vi "Cancel State Machine.vi"   [LabVIEW 2013]
uses:
  typedefs/fg_typedef.ctl
  typedefs/subStates.ctl
  typedefs/singleUseSubstate.ctl
types:
  T1 = typedef "subStates.ctl" = enum16{"null", "wait", "driver control", "auto", "manual override", "hold position", "rotate", "pickup", "pass", "load-shoot", "load-pass", "goto shoot", "shoot", "cancel", "end"}
  T2 = typedef "fg_typedef.ctl" = enum16{"Get", "Set"}
  T3 = typedef "singleUseSubstate.ctl" = enum16{"null", "wait", "shift high", "shift low", "extend shooter", "retract shooter", "close latch", "open latch"}
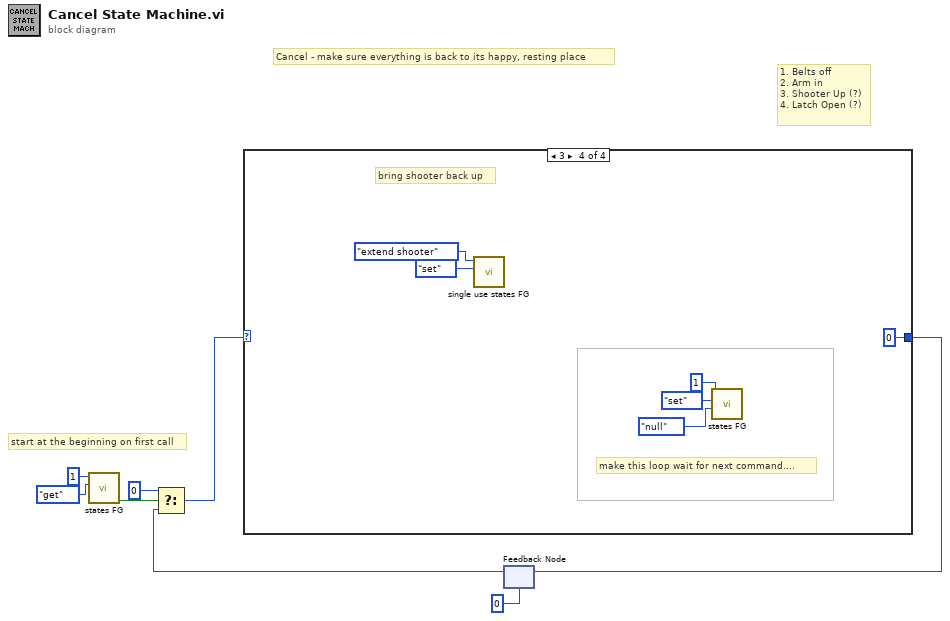
[diagram p0: block diagram]
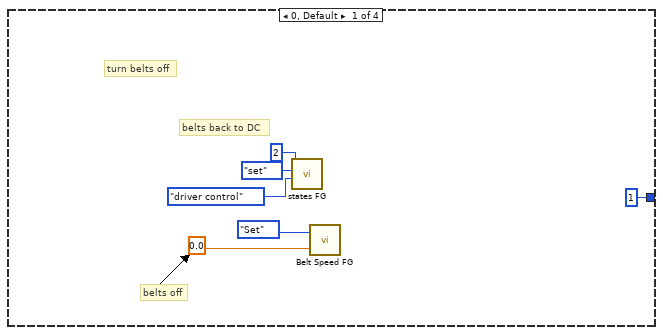
[diagram p2: hidden frame]
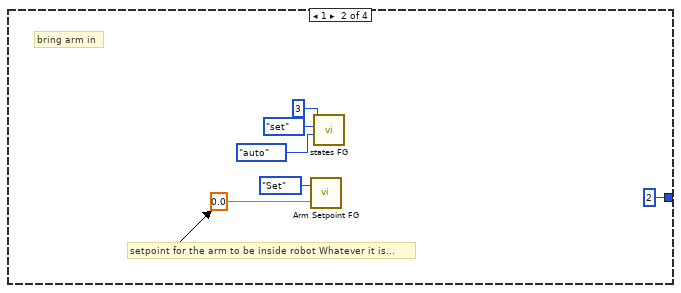
[diagram p3: hidden frame]
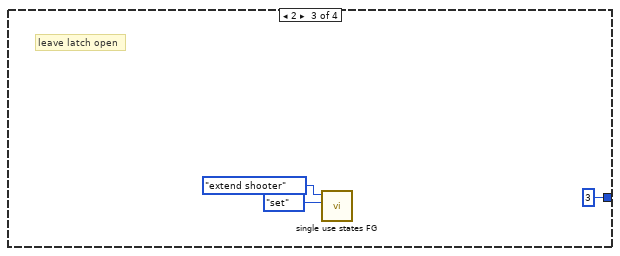
[diagram p4: hidden frame]
diagram:
  # "start at the beginning on first call"
  # "1. Belts off\n2. Arm in\n3. Shooter Up (?)\n4. Latch Open (?)"
  # "Cancel - make sure everything is back to its happy, resting place"
  n1 = call "states FG.vi"("menu (get)"=enum16{"set", "get"}."get", "Loop ID"=1) -> ("first call?"=w1:bool)  [unwired: 6 in, 3 out]
  n2 = feedback #1(0) -> (w4:i32)
  n3 = Select(t=0, s=w1, f=w4) -> (s? t:f=w3:i32)
  n4 = case shown="3" w3 {
    tunnel: [1 2 3 0] -> w7
    frame 0, Default {
      # "belts back to DC"
      # "belts off"
      # "turn belts off"
      n5 = call "states FG.vi"("subState in"=subStates."driver control", "menu (get)"=enum16{"set", "get"}."set", "Loop ID"=2) -> ()  [unwired: 5 in, 4 out]
      n6 = call "Belt Speed FG.vi"("Speed In"=0.0 ("Setpoint In"), "Menu"=fg_typedef."Set") -> ()  [unwired: 1 out]
    }
    frame 1 {
      # "setpoint for the arm to be inside robot Whatever it is..."
      # "bring arm in"
      n7 = call "Arm Setpoint FG.vi"("Setpoint In"=0.0, "Menu"=fg_typedef."Set") -> ()  [unwired: 1 out]
      n8 = call "states FG.vi"("subState in"=subStates."auto", "menu (get)"=enum16{"set", "get"}."set", "Loop ID"=3) -> ()  [unwired: 5 in, 4 out]
    }
    frame 2 {
      # "leave latch open"
      n9 = call "single use states FG.vi"("menu (get)"=enum16{"set", "get"}."set", "substate"=singleUseSubstate."extend shooter") -> ()  [unwired: 6 in, 4 out]
    }
    frame 3 {
      # "make this loop wait for next command...."
      # "bring shooter back up"
      n10 = call "single use states FG.vi"("menu (get)"=enum16{"set", "get"}."set", "substate"=singleUseSubstate."extend shooter") -> ()  [unwired: 6 in, 4 out]
      n11 = call "states FG.vi"("subState in"=subStates."null", "menu (get)"=enum16{"set", "get"}."set", "Loop ID"=1) -> ()  [unwired: 5 in, 4 out]
    }
  }
  n12 = feedback-in #1(w7) -> ()
